vi "DownloadGit.vi"() -> ()   [LabVIEW 2018, in "feGEM DataPacker.lvlib"]
uses:
  <vilib>/WebDAVClient/Simple Get File.vi
  feGEM DataPacker.lvlib
  <vilib>/WebDAVClient/NI_WebDAV.lvlib
panel:
  out "standard error":string
  out "standard output":string
  in  "local file path":path
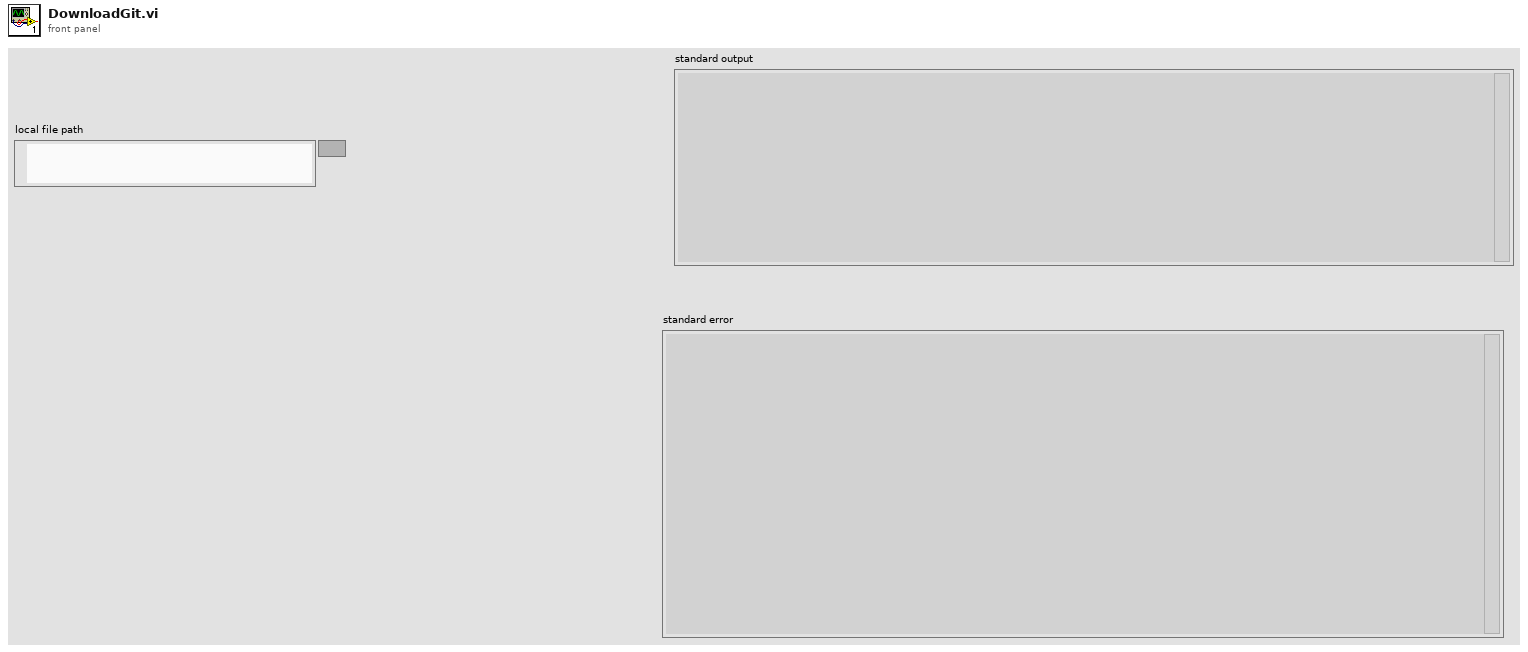
[diagram p1: front panel]
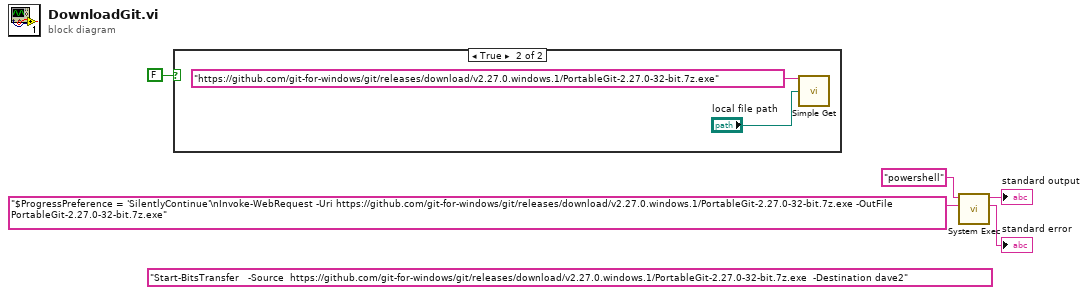
[diagram p0: block diagram]
diagram:
  (unwired) "Start-BitsTransfer   -Source  https://github.com/git-for-windows/git/releases/download/v2.27.0.windows.1/PortableGit-2.27.0-32-bit.7z.exe  -Destination dave2"
  n1 = case shown="True" FALSE {
    frame False {
    }
    frame True {
      n2 = call-poly <vilib>:"Simple Get.vi"("remote file uri"="https://github.com/git-for-windows/git/releases/download/v2.27.0.windows.1/PortableGit-2.27.0-32-bit.7z.exe" ("url"), "local file path"="local file path") -> ()  [unwired: 12 in, 2 out]
    }
  }
  n3 = call <vilib>:"System Exec.vi"("standard input"="$ProgressPreference = 'SilentlyContinue'\nInvoke-WebRequest -Uri https://github.com/git-for-windows/git/releases/download/v2.27.0.windows.1/PortableGit-2.27.0-32-bit.7z.exe -OutFile PortableGit-2.27.0-32-bit.7z.exe" ("command line"), "command line"="powershell") -> ("standard error"=→"standard error":string, "standard output"=→"standard output":string)  [unwired: 6 in, 2 out]
